vi "Panel Resized.vi"(6 "Sizing Refnums 2":T2, 8 "error in (no error)":errorcluster, 9 "Origin":cluster{"H":i16, "V":i16}, 10 "NewBnds":T1={"Left"=0, "Top"=0, "Right"=1280, "Bottom"=720}, 11 "Size Constraints":cluster{"min tab width":i32, "w/h":dbl}={"min tab width"=491, "w/h"=1.333}) -> (0 "error out":errorcluster)   [LabVIEW 2019]
uses:
  <vilib>/Utility/miscctls.llb/LVRectTypeDef.ctl
panel:
  out "WIDTH":dbl
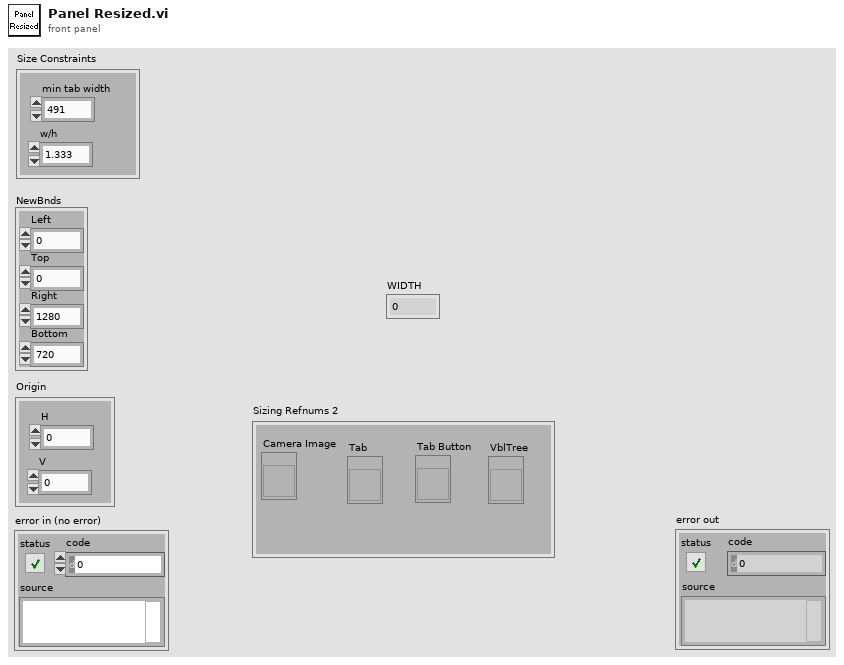
[diagram p1: front panel]
types:
  T1 = typedef "LVRectTypeDef.ctl" = cluster{"Left":i16, "Top":i16, "Right":i16, "Bottom":i16}
  T2 = cluster{"Camera Image":refnum<vi>, "Tab":refnum<vi>, "Tab Button":refnum<vi>, "VblTree":refnum<vi>}
  T3 = typedef "LVPositionTypeDef.ctl" = cluster{"Left":i32, "Top":i32}
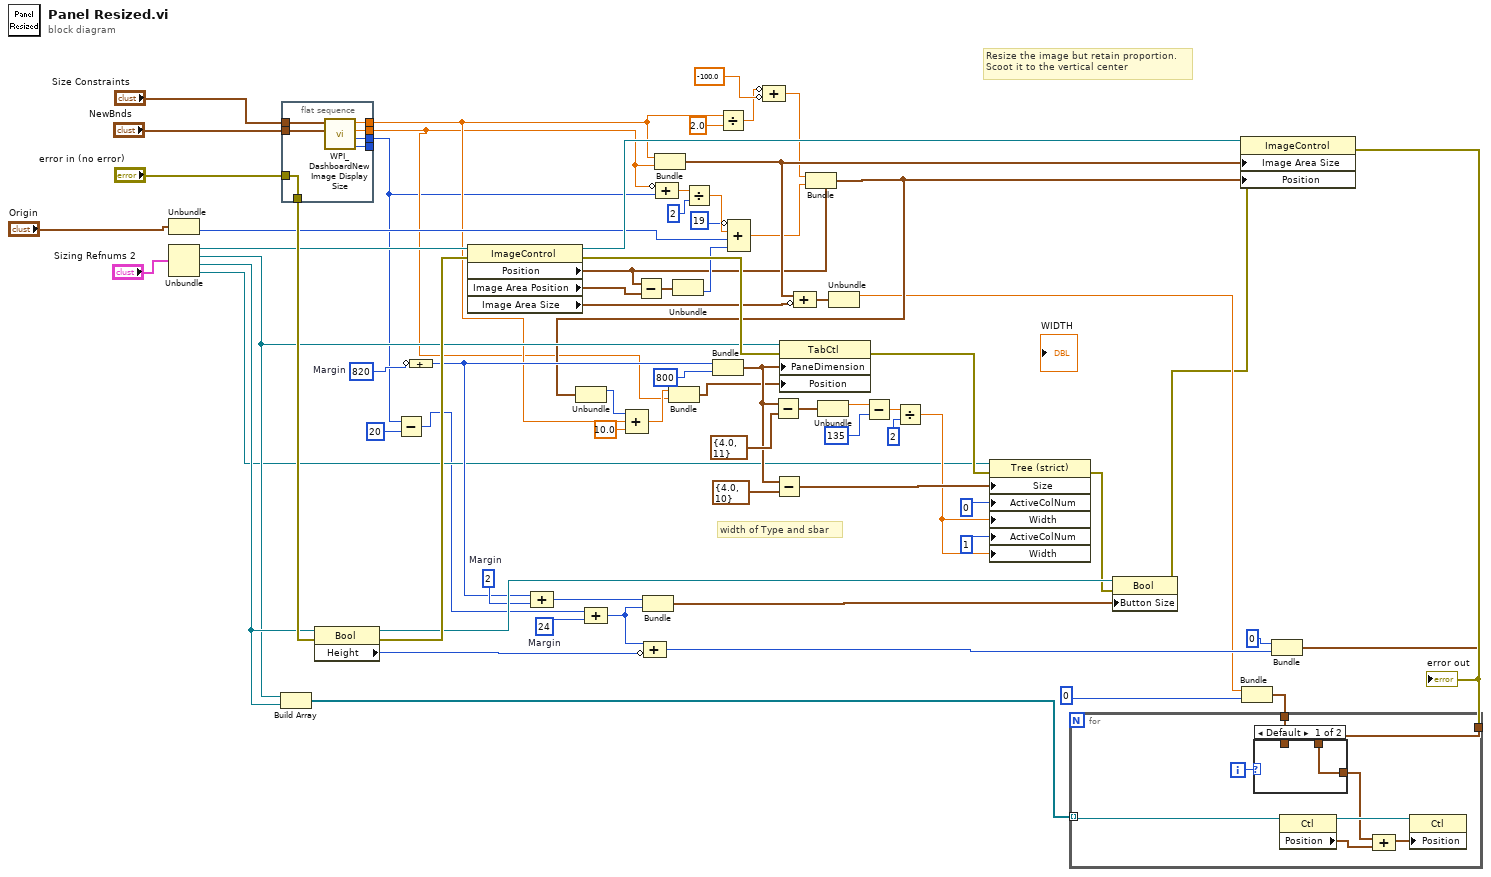
[diagram p0: block diagram]
diagram:
  w65 = 24  # Margin
  w64 = 2  # Margin
  w7 = 820  # Margin
  # "width of Type and sbar"
  # "Resize the image but retain proportion.\nScoot it to the vertical center"
  n1 = Unbundle("Origin") -> ("V"=w46:i16)  [unwired: 1 out]
  n2 = Unbundle("Sizing Refnums 2") -> ("Camera Image"=w40:refnum<vi>, "Tab"=w41:refnum<vi>, "Tab Button"=w48:refnum<vi>, "VblTree"=w21:refnum<vi>)
  n3 = Build Array(w41, w48) -> (w73:refnum<vi>[])
  n4 = flat-sequence {
    tunnel: "NewBnds" -> [w80]
    tunnel: "Size Constraints" -> [w79]
    tunnel: [w78] -> _
    tunnel: [w77] -> w6
    tunnel: [w76] -> w4
    tunnel: [w75] -> w9
    tunnel: [w74] -> w72
    tunnel: "error in (no error)" -> [w74]
    frame #0 {
      n5 = call <vilib>:"WPI_DashboardNew Image Display Size.vi"("NewBnds"=w80, "Size Constraints"=w79) -> ("Window Width"=w78:i16, "Window Height"=w76:i16, "Height"=w77:dbl, "Width"=w75:dbl)  [unwired: 6 in]
    }
  }
  n6 = property class="Bool"(reference=w48, error in=w72) -> (reference out=w68:refnum<vi>, error out=w71:errorcluster, "Height"=w67:u32)
  n7 = Subtract(x=w4, y=i16 20) -> (x-y=w3:i16)
  n8 = Compound Arithmetic op=unknown(invert w7) -> (w63:i32)
  n9 = property class="ImageControl"(reference=w40, error in=w71) -> (reference out=w55:refnum<vi>, error out=w70:errorcluster, "Position"=w54:T3, "Image Area Position"=w50:cluster{"Left":i32, "Top":i32}, "Image Area Size"=w59:cluster{"Width":u32, "Height":u32})
  n10 = Compound Arithmetic op=unknown(w63, w64) -> (w62:i32)
  n11 = Compound Arithmetic op=unknown(w3, w65) -> (w66:i32)
  n12 = Subtract(x=w54, y=w50) -> (x-y=w56:T3)
  n13 = Bundle(w62, w66) -> (w61:cluster{i32, i32})  [unwired: 1 in]
  n14 = Compound Arithmetic op=ADD(w66, invert w67) -> (w25:u32)
  n15 = Bundle("Width"=w9, "Height"=w6) -> (w58:cluster{"Width":dbl, "Height":dbl})  [unwired: 1 in]
  n16 = Compound Arithmetic op=ADD(invert w6, w4) -> (w51:dbl)
  n17 = Unbundle(w56) -> ("Top"=w57:i32)  [unwired: 1 out]
  n18 = Divide(x=w51, y=2) -> (x/y=w53:dbl)
  n19 = Bundle("Margin"=w63, 800) -> (w26:cluster{"Margin":i32, i32})  [unwired: 1 in]
  n20 = Divide(x=w9, y=2.0) -> (x/y=w16:dbl)
  n21 = Compound Arithmetic op=ADD(invert 19, w53, w46, w57) -> (w19:dbl)
  n22 = Compound Arithmetic op=ADD(invert w16, invert -100.0 ("value")) -> (w15:dbl)
  n23 = Subtract(x=w26, y=cluster{dbl, i32} {4.0, 11}) -> (x-y=w34:cluster{dbl, i32})
  n24 = Subtract(x=w26, y=cluster{dbl, i32} {4.0, 10}) -> (x-y=w37:cluster{dbl, i32})
  n25 = Compound Arithmetic op=ADD(w58, invert w59) -> (w60:cluster{"Width":dbl, "Height":dbl})
  n26 = Bundle(cluster=w54, "Left"=w15, "Top"=w19) -> (w14:T3)
  n27 = Unbundle(w14) -> ("Left"=w12:i32)  [unwired: 1 out]
  n28 = Compound Arithmetic op=ADD(w12, w9, 10.0 ("value")) -> (w11:dbl)
  n29 = Bundle(w11, "Height"=w6) -> (w13:cluster{dbl, "Height":dbl})  [unwired: 1 in]
  n30 = property class="TabCtl"(reference=w41, error in=w70, "PaneDimension"=w26, "Position"=w13) -> (error out=w22:errorcluster)  [unwired: 1 out]
  n31 = Unbundle(w34) -> (w33:dbl)  [unwired: 1 out]
  n32 = Unbundle(w60) -> ("Width"=w10:dbl)  [unwired: 1 out]
  n33 = Subtract(x=w33, y=135 ("Active Cell:Active Column Number")) -> (x-y=w30:dbl)
  n34 = Divide(x=w30, y=2 ("Active Cell:Active Column Number")) -> (x/y=w24:dbl)
  n35 = property class="Tree (strict)"(reference=w21, error in=w22, "Size"=w37, "ActiveColNum"=0 ("Active Cell:Active Column Number"), "Width"=w24, "ActiveColNum"=1 ("Active Cell:Active Column Number"), "Width"=w24) -> (error out=w36:errorcluster)  [unwired: 1 out]
  n36 = property class="Bool"(reference=w68, error in=w36, "Button Size"=w61) -> (error out=w5:errorcluster)  [unwired: 1 out]
  n37 = property class="ImageControl"(reference=w55, error in=w5, "Image Area Size"=w58, "Position"=w14) -> (error out=w45:errorcluster)  [unwired: 1 out]
  "error out" <- w45
  n38 = Bundle("Width"=w10, 0) -> (w49:cluster{"Width":dbl, i32})  [unwired: 1 in]
  n39 = Bundle(0, w25) -> (w27:cluster{i32, u32})  [unwired: 1 in]
  n40 = for {
    tunnel: w73 -> [w88] mode=indexing
    tunnel: w49 -> [w83]
    tunnel: w45 -> [_]
    tunnel: w27 -> [w82]
    i -> [w84]
    n41 = case shown="Default" w84 {
      tunnel: w83 -> [_ w90]
      tunnel: w82 -> [w89 _]
      tunnel: [w89 w90] -> w81
      frame Default {
      }
      frame 0, 1 {
      }
    }
    n42 = property class="Ctl"(reference=w88) -> (reference out=w87:refnum<vi>, "Position"=w86:T3)  [unwired: 1 in, 1 out]
    n43 = Compound Arithmetic op=ADD(w81, w86) -> (w85:cluster{dbl, u32})
    n44 = property class="Ctl"(reference=w87, "Position"=w85) -> ()  [unwired: 1 in, 2 out]
  }
